vi "SineWave PID Tune.vi"() -> ()   [LabVIEW 2017]
uses:
  <vilib>/Platform/TimedLoop/XDataNode/timing_clust.ctl
  <vilib>/Platform/TimedLoop/XDataNode/nitl_modes.ctl
  <vilib>/Platform/TimedLoop/XDataNode/wakeup.ctl
  <vilib>/Platform/TimedLoop/XDataNode/XDataNode.xnode
  <vilib>/Platform/TimedLoop/XDataNode/XDNodeRunTimeDep.lvlib
panel:
  out "Mea":dbl
  out "u":dbl
  out "Input":i16
  in  "ENC":i32
  out "Ref":dbl
  out "Input":dbl[](graph)
  in  "Ki":dbl
  in  "Kd":dbl
  in  "Kp":dbl
  in  "사인파 진폭 (M)":dbl
  in  "사인파 주기(f)":dbl
  out "Reference & Measurement":dbl[][](graph)
  in  "정지":bool
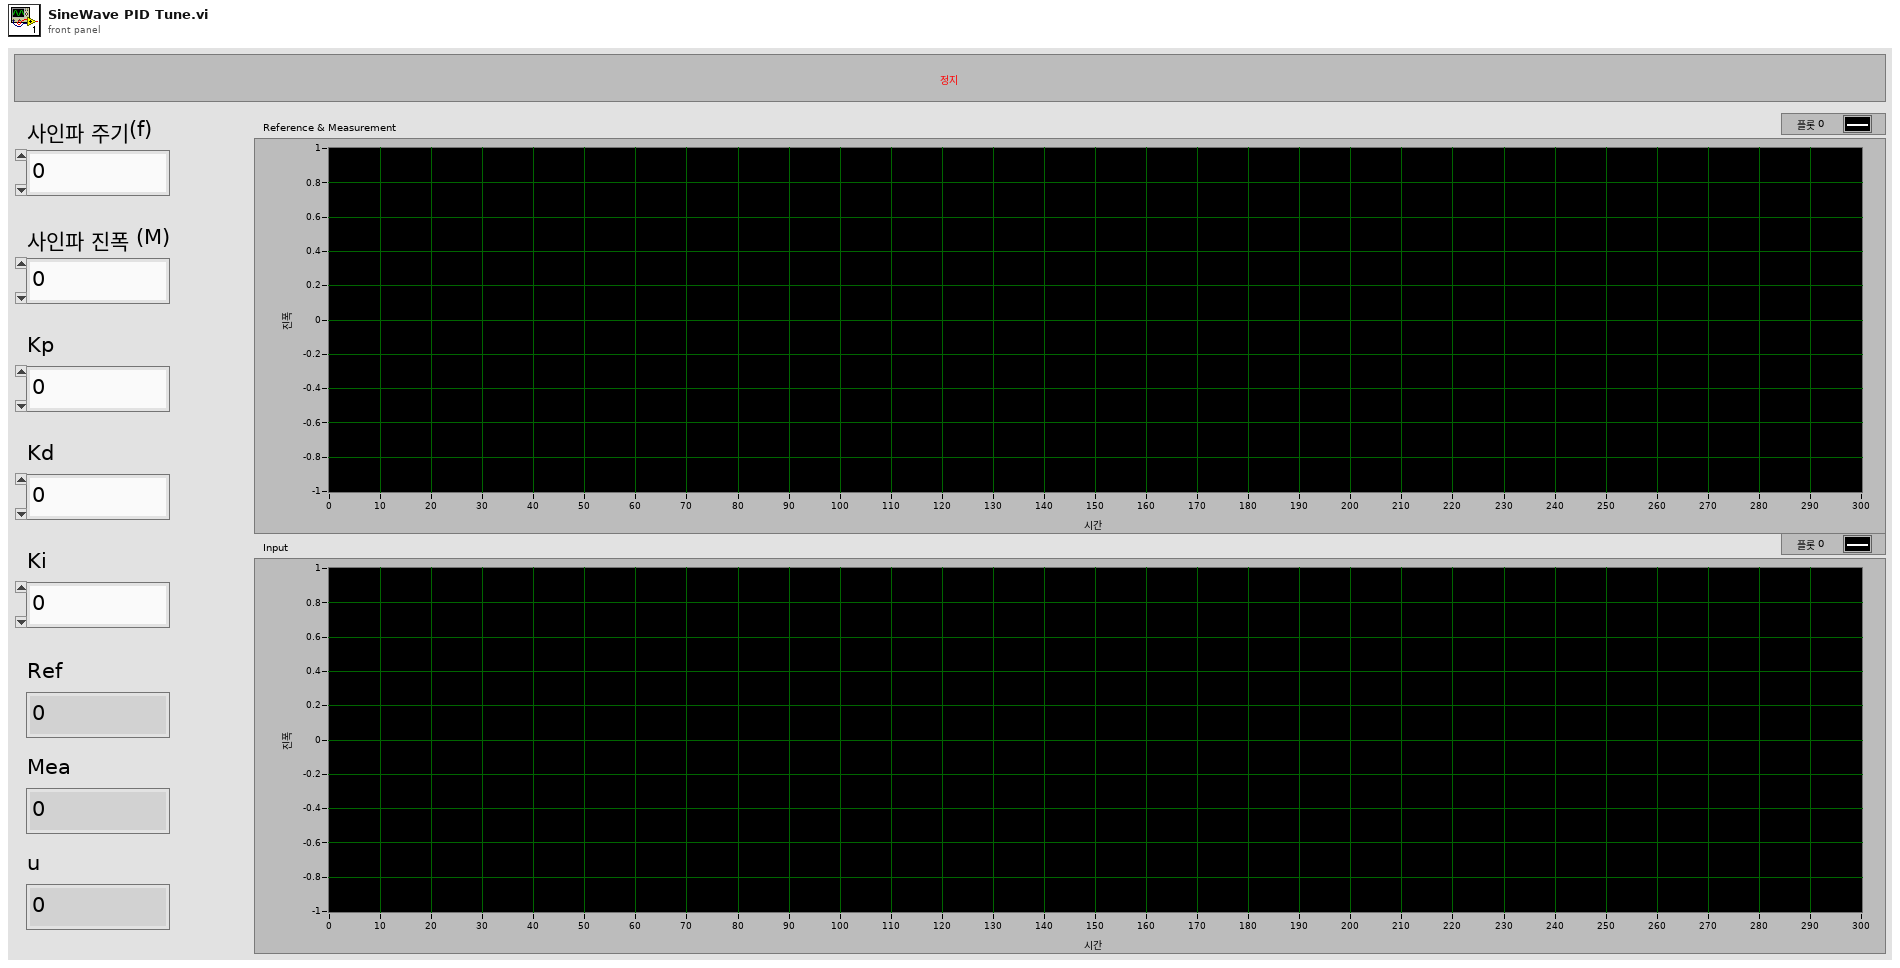
[diagram p1: front panel]
types:
  T1 = typedef "XDNodeRunTimeDep.lvlib/timing_clust.ctl" = cluster{"Expected End [f-1]":u64, "Actual End [f-1]":u64, "Finished Late? [f-1]":bool, "Expected End [i-1]":u64, "Actual End [i-1]":u64, "Finished Late? [i-1]":bool, "Expected Start [i]":u64, "Actual Start [i]":u64, "Expected Start [f]":u64, "Actual Start [f]":u64, "Source Name":string, "Structure Name":string, "Period":i64, "Deadline":i64, "Offset":i64, "Start":i64, "Priority":i32, "Timeout":i32, "Mode":T2, "Wakeup Reason":T3, "Error":errorcluster, "Source Type":string, "Secondary Source Type":string, "Global End Time":u64, "Global Start Time":u64, "Frame Duration":u64, "Iteration Duration":u64, "Assigned CPU":i32, "I/O Scan Engine Mode":u32}
  T2 = typedef "XDNodeRunTimeDep.lvlib/nitl_modes.ctl" = enum32{"No Change", "Process missed periods, maintain original phase", "Discard missed periods, maintain original phase", "Process missed periods, ignore original phase", "Discard missed periods, ignore original phase"}
  T3 = typedef "XDNodeRunTimeDep.lvlib/wakeup.ctl" = enum32{"Normal", "Aborted", "Asynchronous wakeup", "Timing source error", "Timed loop error", "Timeout"}
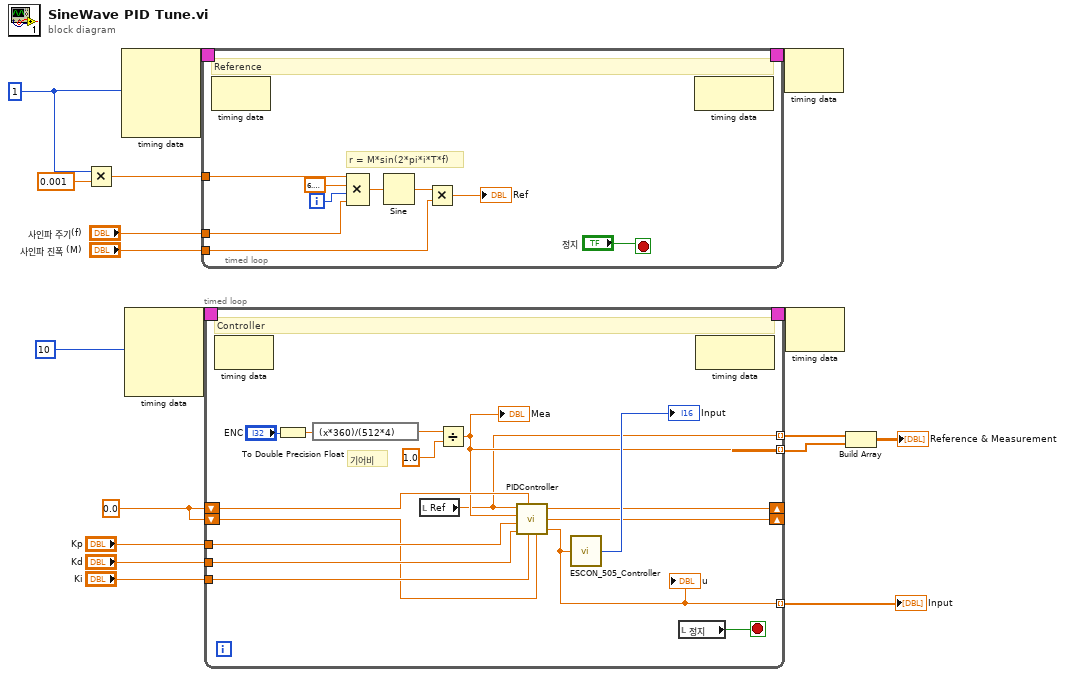
[diagram p0: block diagram]
diagram:
  w5 = 0.0 ("e")
  w16 = i64 1 ("주기")
  n1 = Multiply(x=w16, y=0.001) -> (x*y=w14:dbl)
  n2 = node-c288(w16) -> (w18:T1)  [unwired: 3 in]
  n3 = node-c288(i64 10 ("주기")) -> (w13:T1)  [unwired: 3 in]
  n4 = timed-loop {
    timing: w18 -> [_]
    timing-out: [_] -> w17
    tunnel: w14 -> [w24]
    tunnel: "사인파 주기(f)" -> [w20]
    tunnel: "사인파 진폭 (M)" -> [w19]
    i -> [w21]
    stop <- "정지" stop-if-true
    # "r = M*sin(2*pi*i*T*f)"
    # "Reference"
    n5 = node-c288() -> ()  [unwired: 1 in, 1 out]
    n6 = Compound Arithmetic op=MULTIPLY(w24, 6.283185307179586, w21, w20) -> (w25:dbl)
    n7 = Sine(x=w25) -> (sin(x)=w26:dbl)
    n8 = Multiply(x=w26, y=w19) -> (x*y=→"Ref":dbl)
    n9 = node-c288() -> ()  [unwired: 1 in, 1 out]
  }
  n10 = timed-loop {
    timing: w13 -> [_]
    timing-out: [_] -> w12
    tunnel: "Kp" -> [w33]
    tunnel: "Kd" -> [w34]
    tunnel: "Ki" -> [w35]
    shift-right: [w38] -> _
    shift-left: w5 -> [w39]
    shift-right: [w37] -> _
    shift-left: w5 -> [w30]
    tunnel: [w31] -> w4 mode=indexing
    tunnel: [w32] -> w2 mode=indexing
    tunnel: [w36] -> w1 mode=indexing
    stop <- w45 stop-if-true
    # "기어비"
    # "Controller"
    n11 = node-c288() -> ()  [unwired: 1 in, 1 out]
    n12 = To Double Precision Float(number="ENC") -> (double precision float=w42:dbl)
    n13 = expression code="(x*360)/(512*4)"(w42) -> (w44:dbl)
    n14 = local read "Ref"() -> (w31:dbl)
    n15 = Divide(x=w44, y=1.0) -> (x/y=w32:dbl)
    "Mea" <- w32
    n16 = call "PIDController.vi"("e_Sum_Old"=w30, "Ki"=w35, "Kd"=w34, "Kp"=w33, "eOld"=w39, "Measurement"=w32, "Reference"=w31) -> ("u"=w36:dbl, "e_Sum"=w37:dbl, "e"=w38:dbl)  [unwired: 1 in]
    "u" <- w36
    n17 = call "ESCON_505_Controller.vi"("u"=w36) -> ("Modified u"=→"Input":i16)
    n18 = local read "정지"() -> (w45:bool)
    n19 = node-c288() -> ()  [unwired: 1 in, 1 out]
  }
  "Input" <- w1
  n20 = node-c288(w17) -> ()  [unwired: 1 out]
  n21 = node-c288(w12) -> ()  [unwired: 1 out]
  n22 = Build Array(w4, w2) -> (→"Reference & Measurement":dbl[][])
